vi "niSE_Open.vi"(8 "error in":errorcluster, 10 "Reset?":bool=TRUE, 11 "Alias":string) -> (0 "error out":errorcluster {"code" format="%.0x"}, 3 "Handle":variant)   [LabVIEW 2015]
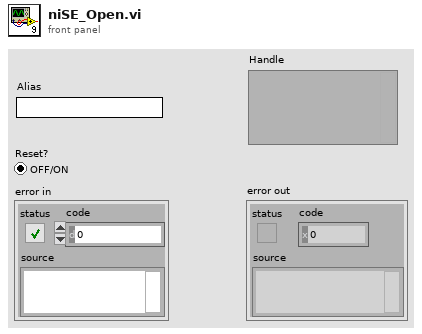
[diagram p1: front panel]
types:
  T1 = typedef "niSE SessionRefnum.ctl" = refnum<k1>
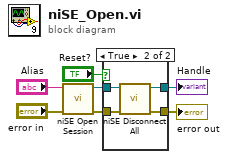
[diagram p0: block diagram]
diagram:
  n1 = call <vilib>:"niSE Open Session.vi"("error in (no error)"="error in", "Virtual Device Name (SwitchConfiguration1)"="Alias") -> ("error out"=w2:errorcluster, "NISE Session (out)"=w4:T1)  [unwired: 4 in]
  n2 = case shown="True" "Reset?" {
    tunnel: w4 -> [w9 w13]
    tunnel: [w9 w12] -> w3
    tunnel: w2 -> [w8 w11]
    tunnel: [w8 w10] -> w1
    frame False {
    }
    frame True {
      n3 = call <vilib>:"niSE Disconnect All.vi"("error in (no error)"=w11, "NISE Session (in)"=w13) -> ("error out"=w10:errorcluster, "NISE Session (out)"=w12:T1)  [unwired: 4 in]
    }
  }
  "Handle" <- w3
  "error out" <- w1
